vi "Sin_wave_graph.vi"() -> ()   [LabVIEW 2022 SP3]
panel:
  out "Waveform Chart":dbl(graph)
  in  "Step":dbl
  out "Iteration":i32
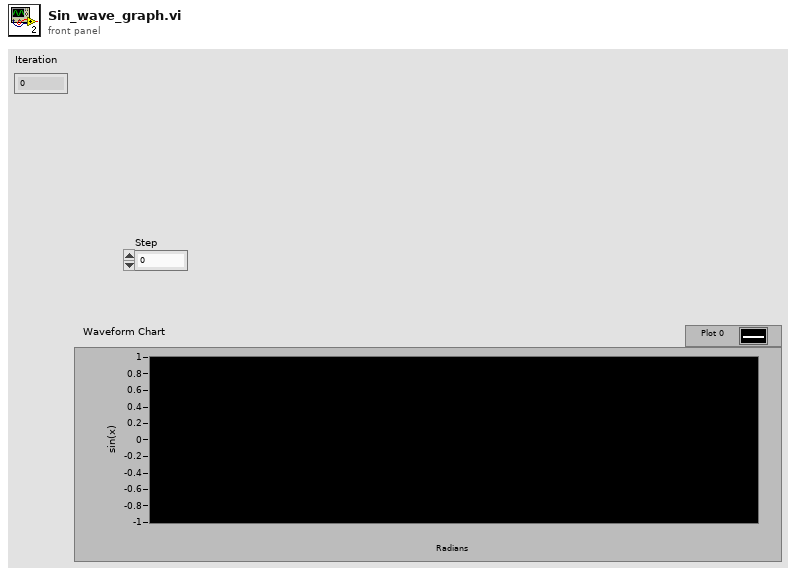
[diagram p1: front panel]
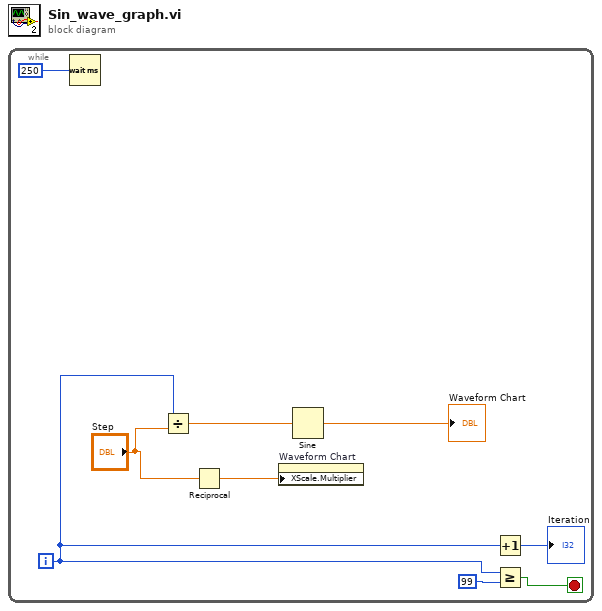
[diagram p0: block diagram]
diagram:
  n1 = while {
    i -> [w5]
    stop <- w8 stop-if-true
    n2 = Wait (ms)(milliseconds to wait=250) -> ()  [unwired: 1 out]
    n3 = Divide(x=w5, y="Step") -> (x/y=w4:dbl)
    n4 = Reciprocal(x="Step") -> (1/x=w2:dbl)
    n5 = property on="Waveform Chart" class="WFChart (strict)"("XScale.Multiplier"=w2) -> ()  [unwired: 2 in, 2 out]
    n6 = Sine(x=w4) -> (sin(x)=→"Waveform Chart":dbl)
    n7 = Increment(x=w5) -> (x+1=→"Iteration":i32)
    n8 = Greater Or Equal?(x=w5, y=99) -> (x >= y?=w8:bool)
  }
